vi "Write to Log File.vi"(1 "error in":errorcluster) -> (0 "error out":errorcluster)   [LabVIEW 2016]
uses:
  Refname/Sensors.ctl
  Refname/Queues.ctl
  Refname/Refname to String (Sensors).vi
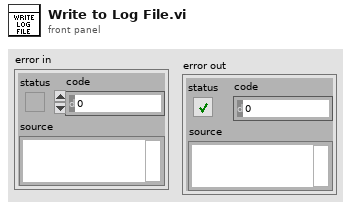
[diagram p1: front panel]
types:
  T1 = typedef "Queues.ctl" = enum16{"Log Queue"}
  T2 = typedef "Sensors.ctl" = enum16{"DIP 1", "DIP 2", "DIP 3", "DIP 4", "IMU", "HuskieBoard"}
  T3 = typedef "WPI_SerialPortRef.ctl" = cluster{"DevStatus":errorcluster, "Serial Port Name":refnum<visa-resource-name>}
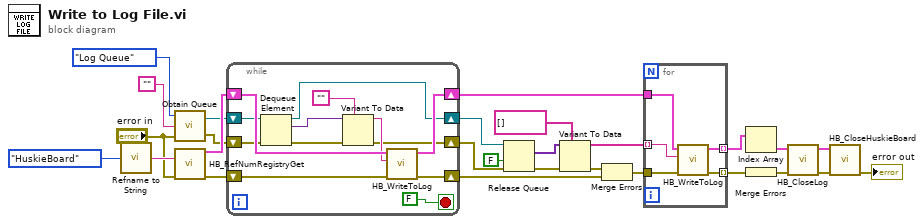
[diagram p0: block diagram]
diagram:
  n1 = call-poly "Refname to String.vi"("Enum"=Sensors."HuskieBoard") -> ("String"=w26:string)
  n2 = call "Obtain Queue.vi"("error in"="error in", "data type"="", "Queue"=Queues."Log Queue") -> ("error out"=w16:errorcluster, "Queue Ref"=w19:refnum<queue>)
  n3 = call <vilib>:"HB_RefNumRegistryGet.vi"("refnum name"=w26, "error in (no error)"="error in") -> ("HBDevRef"=w23:T3, "error out"=w22:errorcluster)  [unwired: 12 in]
  n4 = while {
    shift-right: [w39] -> w6
    shift-left: w23 -> [w40]
    shift-right: [w36] -> w15
    shift-left: w19 -> [w37]
    shift-right: [w38] -> w7
    shift-left: w22 -> [w33]
    shift-right: [w28] -> w13
    shift-left: w16 -> [w29]
    stop <- FALSE stop-if-true
    n5 = Dequeue Element(queue=w37, error in (no error)=w29) -> (queue out=w36:refnum<queue>, element=w35:variant, error out=w30:errorcluster)  [unwired: 1 in, 1 out]
    n6 = Variant To Data(error in=w30, type="", Variant=w35) -> (data=w32:string, error out=w28:errorcluster)
    n7 = call <vilib>:"HB_WriteToLog.vi"("error in (no error)"=w33, "Log string"=w32, "HBDevRef"=w40) -> ("error out"=w38:errorcluster, "HBDevRef"=w39:T3)  [unwired: 7 in]
  }
  n8 = Release Queue(queue=w15, force destroy? (F)=FALSE, error in (no error)=w13) -> (remaining elements=w12:variant[], error out=w11:errorcluster)  [unwired: 1 out]
  n9 = Variant To Data(error in=w11, type=string[] [], Variant=w12) -> (data=w9:string[], error out=w8:errorcluster)
  n10 = Merge Errors(w8, w7) -> (w3:errorcluster)
  n11 = for {
    tunnel: w9 -> [w45] mode=indexing
    tunnel: w6 -> [w44]
    tunnel: [w43] -> w5 mode=indexing
    tunnel: w3 -> [w42]
    tunnel: [w41] -> w2 mode=indexing
    n12 = call <vilib>:"HB_WriteToLog.vi"("error in (no error)"=w42, "Log string"=w45, "HBDevRef"=w44) -> ("error out"=w41:errorcluster, "HBDevRef"=w43:T3)  [unwired: 7 in]
  }
  n13 = Index Array(array=w5) -> (element=w4:T3)  [unwired: 1 in]
  n14 = Merge Errors(w2) -> (w1:errorcluster)
  n15 = call <vilib>:"HB_CloseLog.vi"("error in (no error)"=w1, "HBDeviceRef"=w4) -> ("error out"=w25:errorcluster, "HBDeviceRef"=w24:T3)  [unwired: 8 in]
  n16 = call <vilib>:"HB_CloseHuskieBoard.vi"("error in (no error)"=w25, "HBDeviceRef"=w24) -> ("error out"=→"error out":errorcluster)  [unwired: 9 in]
